vi "Visible IncDec.vi"(8 "error in (no error)":errorcluster, 10 "inc/dec":enum8{"hide", "show"}(ring), 11 "GObject in":refnum<vi>) -> (0 "error out":errorcluster, 1 "was inc/dec visible?":enum8{"hide", "show"}(ring), 2 "has inc/dec?":bool, 3 "GObject out":refnum<vi>)   [LabVIEW 2019, in "Builtins.lvlib"]
doc: "Shows or hides the increment / decrement buttons if it exists.\nNote: Timestamps do not have an available property node to set the buttons visibility(LV2019 bug)\n\nCreated by: Ryan Pacini"
uses:
  Builtins.lvlib
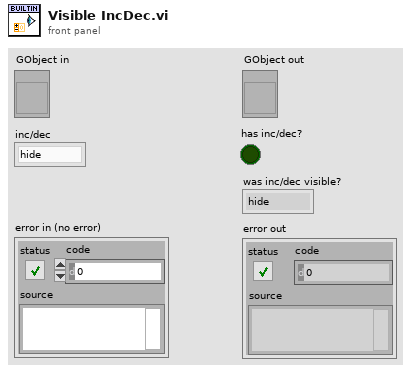
[diagram p1: front panel]
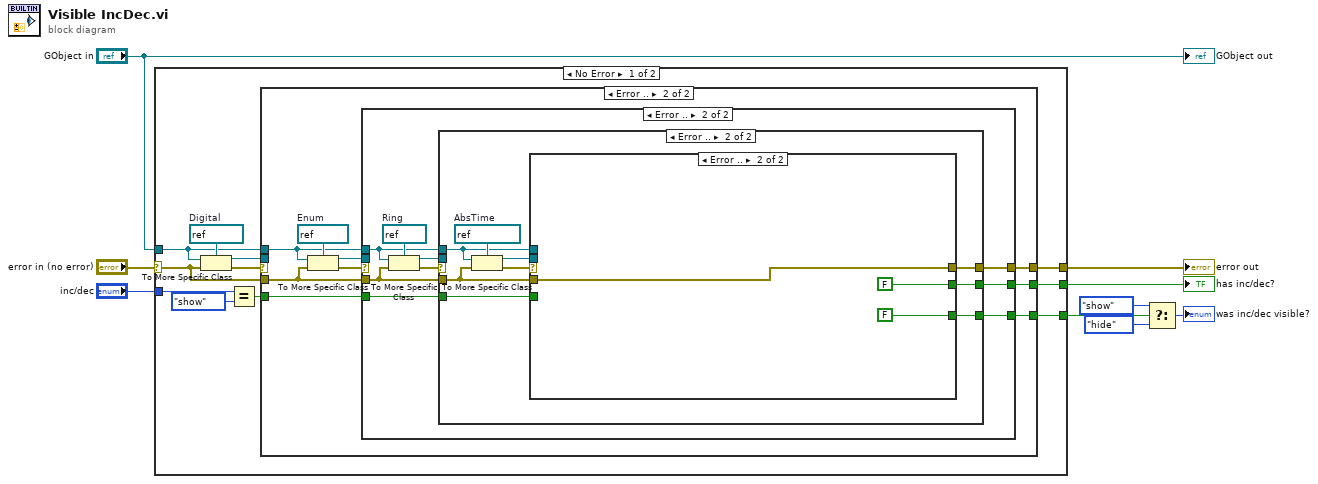
[diagram p0: block diagram]
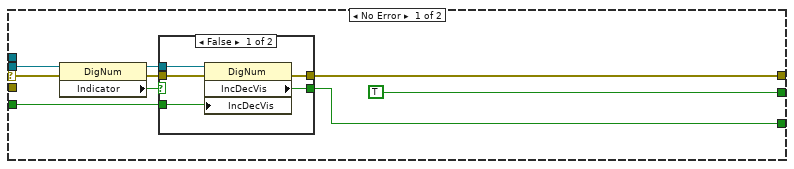
[diagram p2: hidden frame]
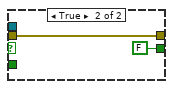
[diagram p3: hidden frame]
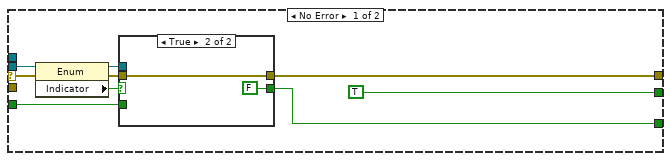
[diagram p4: hidden frame]
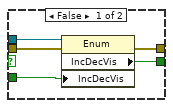
[diagram p5: hidden frame]
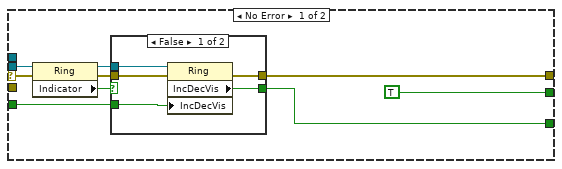
[diagram p6: hidden frame]
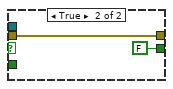
[diagram p7: hidden frame]
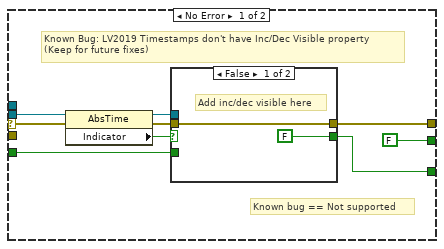
[diagram p8: hidden frame]
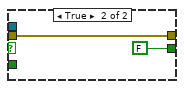
[diagram p9: hidden frame]
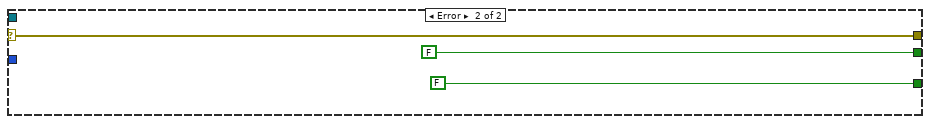
[diagram p10: hidden frame]
diagram:
  n1 = case shown="No Error" "error in (no error)" {
    selector: "error in (no error)" -> [w16 w114]
    tunnel: "GObject in" -> [w18 _]
    tunnel: "inc/dec" -> [w12 _]
    tunnel: [w20 w114] -> w7
    tunnel: [w15 FALSE] -> w6
    tunnel: [w13 FALSE ("ScrollVis")] -> w4
    frame No Error {
      w19 = refnum<vi> refnum  # Digital
      n2 = To More Specific Class(target class=w19, reference=w18, error in=w16) -> (specific class reference=w14:refnum<vi>, error out=w17:errorcluster)
      n3 = Equal?(x=w12, y=enum8{"hide", "show"}."show") -> (x = y?=w10:bool)
      n4 = case shown="Error .." w17 {
        selector: w17 -> [w27 _]
        tunnel: w10 -> [w22 w41]
        tunnel: [w28 w42] -> w20
        tunnel: w18 -> [_ w39]
        tunnel: w16 -> [_ w40]
        tunnel: [TRUE w38] -> w15
        tunnel: w14 -> [w25 _]
        tunnel: [w21 w37] -> w13
        frame No Error {
          n5 = property class="DigNum"(reference=w25, error in=w27) -> (reference out=w24:refnum<vi>, error out=w26:errorcluster, "Indicator"=w23:bool)
          n6 = case shown="False" w23 {
            tunnel: [w34 w36] -> w28
            tunnel: w26 -> [w33 w36]
            tunnel: w24 -> [w32 _]
            tunnel: w22 -> [w31 _]
            tunnel: [w30 FALSE ("IncDecVis")] -> w21
            frame False {
              n7 = property class="DigNum"(reference=w32, error in=w33, "IncDecVis"=w31) -> (error out=w34:errorcluster, "IncDecVis"=w30:bool)  [unwired: 1 out]
            }
            frame True {
            }
          }
        }
        frame Error {
          w45 = refnum<vi> refnum  # Enum
          n8 = To More Specific Class(target class=w45, reference=w39, error in=w40) -> (specific class reference=w43:refnum<vi>, error out=w44:errorcluster)
          n9 = case shown="Error .." w44 {
            selector: w44 -> [w50 _]
            tunnel: w43 -> [w49 _]
            tunnel: [w47 w66] -> w42
            tunnel: w41 -> [w48 w67]
            tunnel: w40 -> [_ w65]
            tunnel: w39 -> [_ w64]
            tunnel: [TRUE w63] -> w38
            tunnel: [w46 w62] -> w37
            frame No Error {
              n10 = property class="Enum"(reference=w49, error in=w50) -> (reference out=w52:refnum<vi>, error out=w53:errorcluster, "Indicator"=w51:bool)
              n11 = case shown="True" w51 {
                tunnel: [w59 w61] -> w47
                tunnel: w53 -> [w58 w61]
                tunnel: w52 -> [w57 _]
                tunnel: w48 -> [w56 _]
                tunnel: [w55 FALSE ("IncDecVis")] -> w46
                frame False {
                  n12 = property class="Enum"(reference=w57, error in=w58, "IncDecVis"=w56) -> (error out=w59:errorcluster, "IncDecVis"=w55:bool)  [unwired: 1 out]
                }
                frame True {
                }
              }
            }
            frame Error {
              w70 = refnum<vi> refnum  # Ring
              n13 = To More Specific Class(target class=w70, reference=w64, error in=w65) -> (specific class reference=w68:refnum<vi>, error out=w69:errorcluster)
              n14 = case shown="Error .." w69 {
                selector: w69 -> [w75 _]
                tunnel: w68 -> [w73 _]
                tunnel: w67 -> [w74 w95]
                tunnel: [w72 w94] -> w66
                tunnel: w65 -> [_ w90]
                tunnel: w64 -> [_ w89]
                tunnel: [TRUE w93] -> w63
                tunnel: [w71 w92] -> w62
                frame No Error {
                  n15 = property class="Ring"(reference=w73, error in=w75) -> (reference out=w77:refnum<vi>, error out=w78:errorcluster, "Indicator"=w76:bool)
                  n16 = case shown="False" w76 {
                    tunnel: [w84 w86] -> w72
                    tunnel: w78 -> [w83 w86]
                    tunnel: w77 -> [w82 _]
                    tunnel: w74 -> [w81 _]
                    tunnel: [w80 FALSE ("IncDecVis")] -> w71
                    frame False {
                      n17 = property class="Ring"(reference=w82, error in=w83, "IncDecVis"=w81) -> (error out=w84:errorcluster, "IncDecVis"=w80:bool)  [unwired: 1 out]
                    }
                    frame True {
                    }
                  }
                }
                frame Error {
                  w91 = refnum<vi> refnum  # AbsTime
                  n18 = To More Specific Class(target class=w91, reference=w89, error in=w90) -> (specific class reference=w87:refnum<vi>, error out=w88:errorcluster)
                  n19 = case shown="Error .." w88 {
                    selector: w88 -> [w101 _]
                    tunnel: w95 -> [w99 _]
                    tunnel: [w98 w111] -> w94
                    tunnel: w90 -> [_ w111]
                    tunnel: [FALSE FALSE] -> w93
                    tunnel: w89 -> [_ _]
                    tunnel: [w96 FALSE ("ScrollVis")] -> w92
                    tunnel: w87 -> [w100 _]
                    frame No Error {
                      # "Known bug == Not supported"
                      # "Known Bug: LV2019 Timestamps don't have Inc/Dec Visible property\n(Keep for future fixes)"
                      n20 = property class="AbsTime"(reference=w100, error in=w101) -> (reference out=w103:refnum<vi>, error out=w104:errorcluster, "Indicator"=w102:bool)
                      n21 = case shown="False" w102 {
                        tunnel: [w106 w108] -> w98
                        tunnel: w104 -> [w106 w108]
                        tunnel: w103 -> [_ _]
                        tunnel: w99 -> [_ _]
                        tunnel: [FALSE ("IncDecVis") FALSE ("IncDecVis")] -> w96
                        frame False {
                          # "Add inc/dec visible here"
                        }
                        frame True {
                        }
                      }
                    }
                    frame Error {
                    }
                  }
                }
              }
            }
          }
        }
      }
    }
    frame Error {
    }
  }
  "error out" <- w7
  "has inc/dec?" <- w6
  n22 = Select(t=enum8{"hide", "show"}."show" ("was inc/dec visible?"), s=w4, f=enum8{"hide", "show"}."hide" ("was inc/dec visible?")) -> (s? t:f=→"was inc/dec visible?":enum8{"hide", "show"})
  "GObject out" <- "GObject in"
